vi "test.vi"() -> ()   [LabVIEW 2017]
uses:
  <vilib>/Analysis/2dsp.llb/Power Spectrum (DBL).vi
  <vilib>/Analysis/3filter.llb/Chebyshev Filter (DBL).vi
  <vilib>/Analysis/NI_AALPro.lvlib
  <vilib>/measure/NI_MABase.lvlib
  <vilib>/Analysis/NI_AALBase.lvlib
panel:
  in  "stop":bool
  in  "fe":dbl=1.0 caption="fréq. d'échantillonnage : fé" format="%0.2f"
  out "Graphe":dbl[](graph)
  out "Table 2":string[][](table) caption="Table"
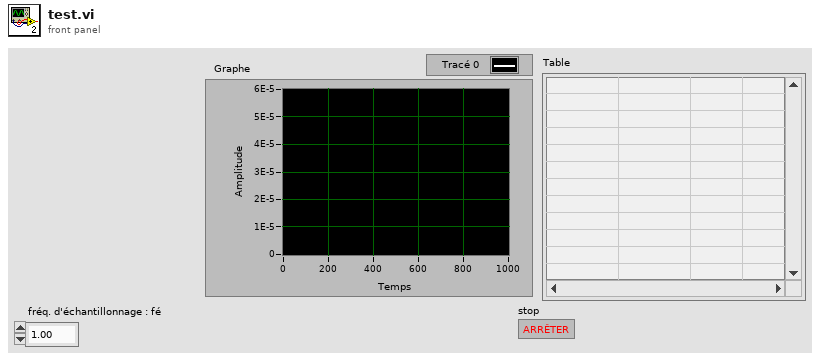
[diagram p1: front panel]
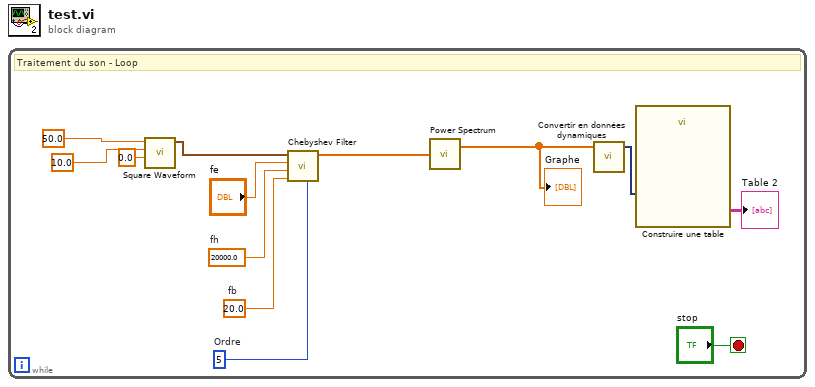
[diagram p0: block diagram]
diagram:
  n1 = while "Boucle While" {
    stop <- "stop" stop-if-true
    w9 = 5  # Ordre
    w10 = 20000.0  # fh
    w11 = 20.0  # fb
    # "Traitement du son - Loop"
    n2 = call <vilib>:"Square Waveform.vi"("phase"=0.0, "amplitude"=10.0, "frequency"=50.0) -> ("signal out"=w5:waveform(dbl))  [unwired: 7 in, 1 out]
    n3 = call-poly <vilib>:"Chebyshev Filter.vi"("order"=w9, "low cutoff freq: fl"=w11, "high cutoff freq: fh"=w10, "sampling freq: fs"="fe", "X"=w5) -> ("Filtered X"=w13:dbl[])  [unwired: 5 in, 1 out]
    n4 = call-poly <vilib>:"Power Spectrum.vi"("X"=w13) -> ("Power Spectrum"=w8:dbl[])  [unwired: 1 out]
    "Graphe" <- w8
    n5 = call "Convertir en données dynamiques"("Array"=w8) -> ("Dynamic Data Type"=w7:dynamicdata)  [unwired: 3 in]
    n6 = call "Construire une table"("Signals"=w7) -> ("Table"=→"Table 2":string[][])  [unwired: 4 in, 6 out]
  }
